vi "Auton_Exist.vi"   [LabVIEW 2019]
uses:
  Robot Global Data.vi
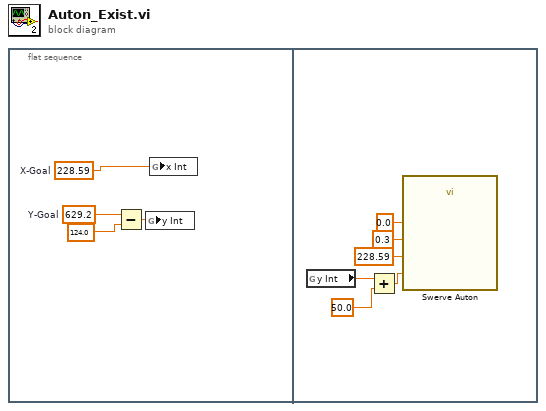
[diagram p0: block diagram]
diagram:
  n1 = flat-sequence {
    frame #0 {
      w4 = 228.59  # X-Goal
      w2 = 629.2  # Y-Goal
      n2 = Subtract(x=w2, y=124.0) -> (x-y=w3:dbl)
      n3 = global write "Robot Global Data.vi" "y Int"(w3) -> ()
      n4 = global write "Robot Global Data.vi" "x Int"(w4) -> ()
    }
    frame #1 {
      n5 = global read "Robot Global Data.vi" "y Int"() -> (w9:dbl)
      n6 = Add(x=w9, y=50.0 ("y Distance")) -> (x+y=w10:dbl)
      n7 = call "Swerve Auton.vi"("Heading"=0.0, "y Distance"=w10, "x Distance"=228.59, "Power"=0.3) -> ()  [unwired: 8 in]
    }
  }
